vi "Auto 6.vi"(8 "Error In":errorcluster) -> (0 "Error Out":errorcluster)   [LabVIEW 2014]
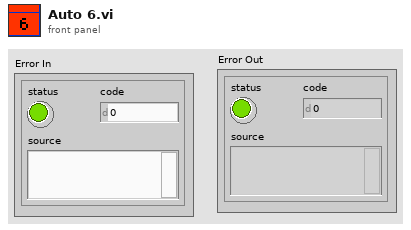
[diagram p1: front panel]
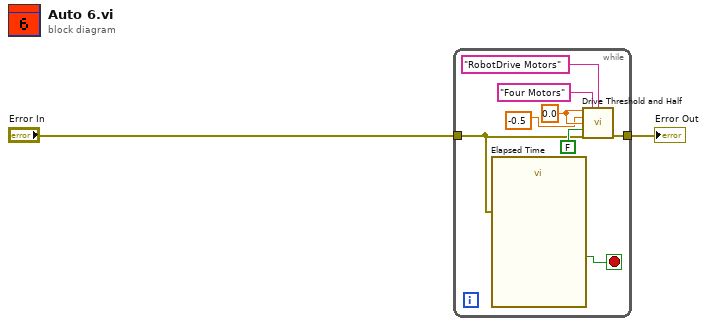
[diagram p0: block diagram]
diagram:
  n1 = while {
    tunnel: "Error In" -> [w3]
    tunnel: [w7] -> w2
    stop <- w4 stop-if-true
    w6 = 0.0 ("Arm Value")
    n2 = call "Elapsed Time"("error in (no error)"=w3) -> ("Time has Elapsed"=w4:bool)  [unwired: 11 in, 7 out]
    n3 = call "Drive Threshold and Half.vi"("X In"=w6, "Drive refnum name"="Four Motors" ("refnum name"), "Send to DB Name"="RobotDrive Motors" ("Name"), "Y In"=-0.5 ("X In"), "R In"=w6, "Speed Toggle"=FALSE ("Grabber Open/Close"), "Error In"=w3) -> ("Error Out"=w7:errorcluster)  [unwired: 8 in]
  }
  "Error Out" <- w2
